vi "read_UI_user_events.vi"(8 "error in (no error)":errorcluster, 11 "panel in":refnum<class "panel.lvclass">) -> (0 "error out":errorcluster, 2 "ui_user_events":T1, 3 "panel out":refnum<class "panel.lvclass">)   [LabVIEW 2015, in "panel.lvclass"]
uses:
  panel.lvclass
  front_panel_class/ui_user_events.ctl
  panel.lvclass/panel.ctl
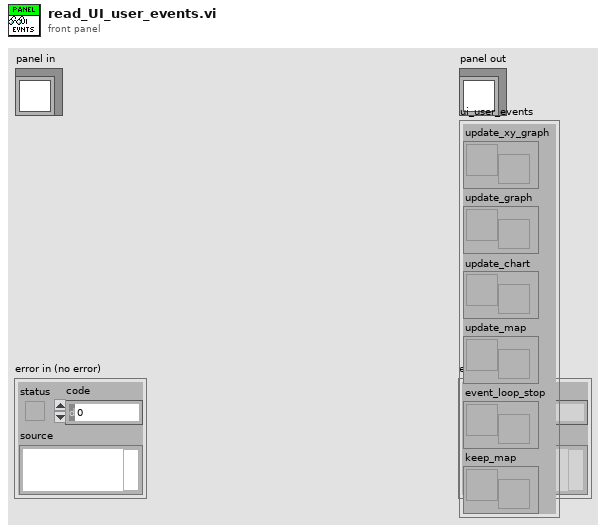
[diagram p1: front panel]
types:
  T1 = typedef "ui_user_events.ctl" = cluster{"update_xy_graph":refnum<user-event>, "update_graph":refnum<user-event>, "update_chart":refnum<user-event>, "update_map":refnum<user-event>, "event_loop_stop":refnum<user-event>, "keep_map":refnum<user-event>}
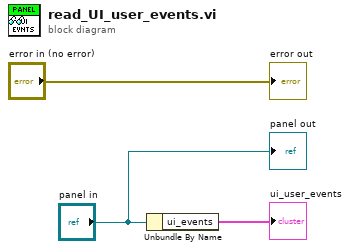
[diagram p0: block diagram]
diagram:
  n1 = Unbundle By Name("panel in") -> ("ui_events"=→"ui_user_events":T1)
  "error out" <- "error in (no error)"
  "panel out" <- "panel in"
